vi "Write operation (0_open).vi"(8 "error in (no error)":errorcluster, 10 "operation (0:open)":T1(ring)=enum."replace or create", 11 "Write_to_file in":refnum<class "Write_to_file.lvclass">) -> (0 "error out":errorcluster, 3 "Write_to_file out":refnum<class "Write_to_file.lvclass">)   [LabVIEW 2015, in "Write_to_file.lvclass"]
uses:
  Write_to_file.lvclass
  Write_to_file.lvclass/Write_to_file.ctl
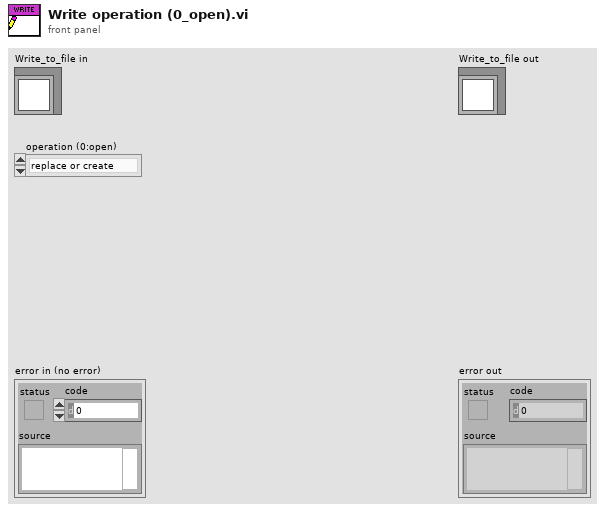
[diagram p1: front panel]
types:
  T1 = enum16{"open", "replace", "create", "open or create", "replace or create", "replace or create with confirmation"}
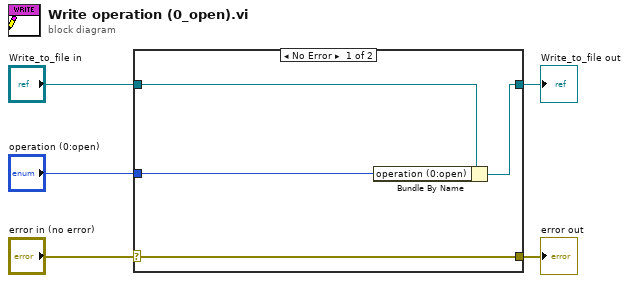
[diagram p0: block diagram]
diagram:
  n1 = case shown="No Error" "error in (no error)" {
    selector: "error in (no error)" -> [w9 w10]
    tunnel: [w9 w10] -> w4
    tunnel: [w7 w11] -> w2
    tunnel: "Write_to_file in" -> [w8 w11]
    tunnel: "operation (0:open)" -> [w6 _]
    frame No Error {
      n2 = Bundle By Name(cluster=w8, "operation (0:open)"=w6) -> (w7:refnum<class "Write_to_file.lvclass">)
    }
    frame Error {
    }
  }
  "error out" <- w4
  "Write_to_file out" <- w2
